vi "LaneExtractorHenes.vi"() -> ()   [LabVIEW 2024]
uses:
  <vilib>/userDefined/High Color/IMAQdx.ctl
  <vilib>/Instr/_visa.llb/VISA Set IO Buffer Mask.ctl
  <vilib>/Instr/_visa.llb/VISA Flush IO Buffer Mask.ctl
  <vilib>/Python/Open Venv Python Session.vi
  <vilib>/Instr/_visa.llb/VISA Configure Serial Port (Instr).vi
  <vilib>/vision/NI_Vision_Development_Module.lvlib
  <vilib>/vision/driver/NI_Vision_Acquisition_Software.lvlib
panel:
  in  "File Path":path=path "C:/Users/JungiHong/OneDrive/Hongik/HI-RACE/2026-01/ExperimentModules/LaneTracking/sampleImages/KakaoTalk_20260312_120930048.jpg"
  in  "UseVideo":bool
  in  "Cam No.":T1="cam3"
  out "Debug":T2(plugin-control)
  in  "input_spd":i16
  in  "HENES":refnum<visa-resource-name>="COM5"
  out "E-STOP":bool
  out "Remote_M/A":bool
  out "Steer_Feed":dbl
  out "Alive_PCU":u8(slide) scale=0.0..254.0
  out "Gear_Feed":u8
  out "Speed_Feed(RPM)":dbl format="%#_g rpm"
  out "버퍼 읽기":string
  out "Speed_Feed(m/s)":dbl
  in  "HLV_Gear":u8
  in  "HLV_A/M":bool=TRUE
  in  "HLV_E-stop":bool
  out "HENES Loop Time":u32=19
  in  "v(Velocity)m/s":dbl=1.0
  in  "k(Gain)":dbl=1.0
  out "δ(OutputSteer)degrees":dbl=17.662742890531817
  in  "max_rmse":u32=1000
  in  "min_span":u32=4
  in  "min_area":u32=4
  out "Right":T2(plugin-control)
  out "B":u8[][](array[numeric])
  out "G":u8[][](array[numeric])
  out "R":u8[][](array[numeric])
  out "changearray":u32=6
  out "CV Loop Time":u32=134
  out "error out 2":errorcluster
  out "error out":errorcluster
  out "return value":string[](array[string])=["0.0", "0.31842436928828866", "C:\\Users\\JungiHong\\OneDrive\\Hongik\\HI-RACE\\2026-01\\ExperimentModules\\LaneTracking\\DebugImageFolder\\left_lane.png", "C:\\Users\\JungiHong\\OneDrive\\Hongik\\HI-RACE\\2026-01\\ExperimentModules\\LaneTracking\\DebugImageFolder\\right_lane.png", "C:\\Users\\JungiHong\\OneDrive\\Hongik\\HI-RACE\\2026-01\\ExperimentModules\\LaneTracking\\DebugImageFolder\\debug_image.png"]
  out "python_error":errorcluster
  out "Left":T2(plugin-control)
  in  "stop":bool
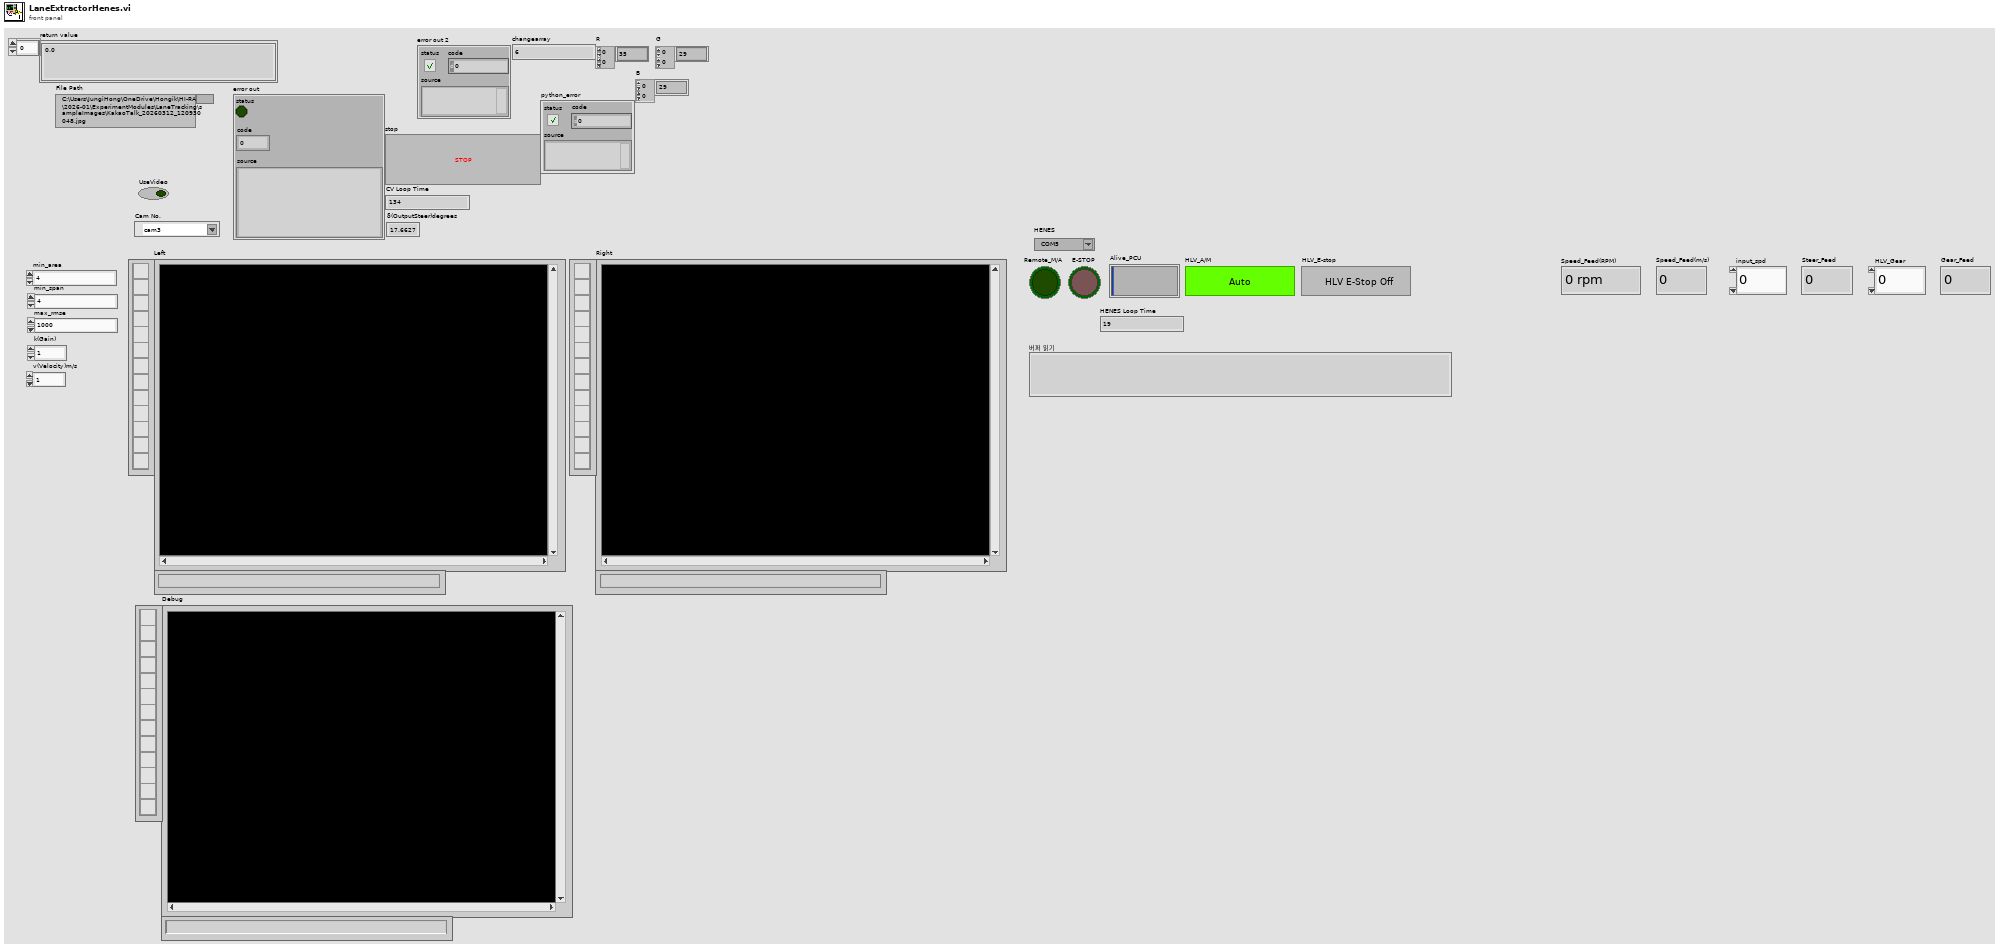
[diagram p1: front panel]
types:
  T1 = typedef "IMAQdx.ctl" = refnum<k21>
  T2 = typedef "IMAQ Image.ctl" = refnum<image>
  T3 = cluster{"HENES_M/A":u8, "HENES_E-Stop":u8, "HENES_Gear":u8, "HENES_Speed":i16, "HENES_Steer":i16, "HENES_Alive":u8}
  T4 = typedef "VISA Flush IO Buffer Mask.ctl" = u16
  T5 = typedef "VISA Set IO Buffer Mask.ctl" = u16
  T6 = cluster{"HLV_M/A_Status":u8, "HLV_E-Stop":u8, "HLV_Gear":u8, "HLV_Speed":i16, "HLV_Steer":i16, "HLV_Alive":u8}
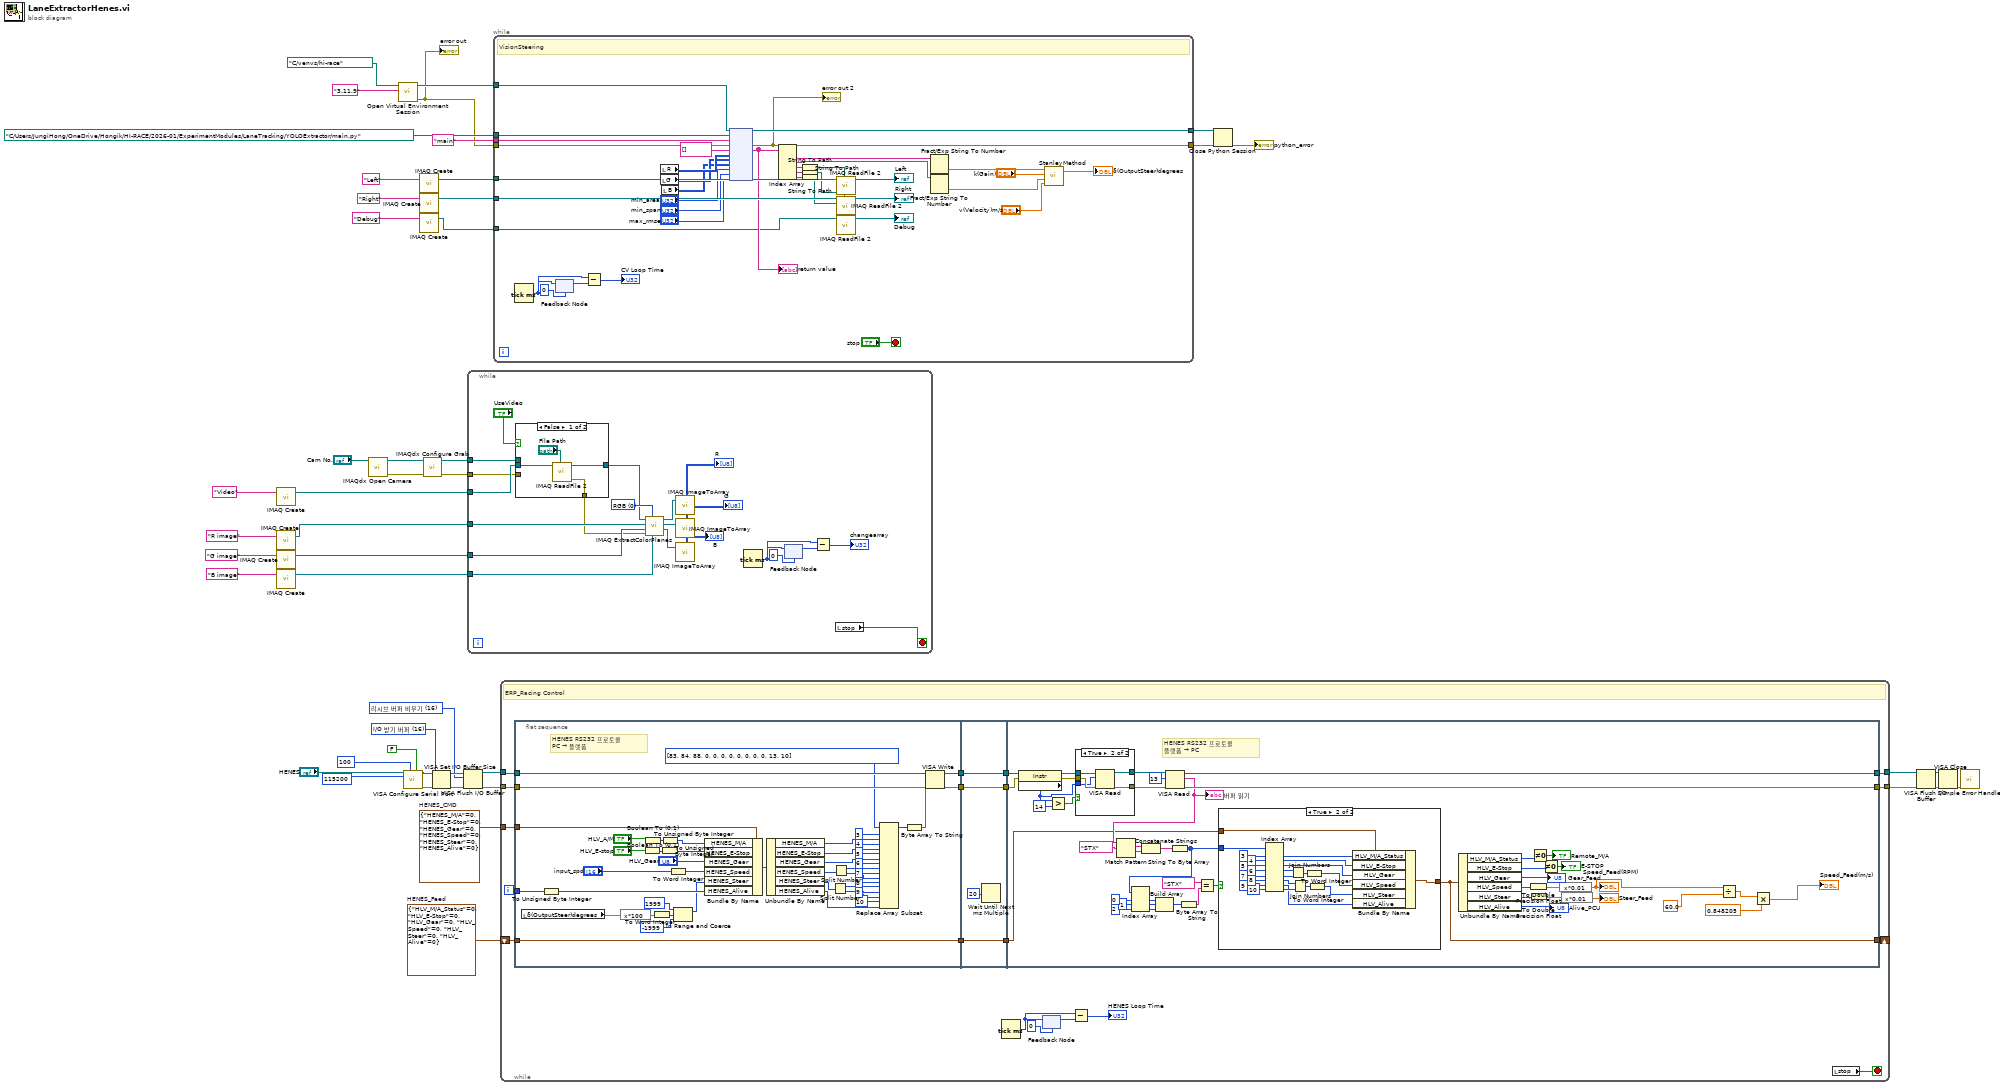
[diagram p0: block diagram]
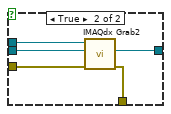
[diagram p4: hidden frame]
diagram:
  w9 = T3 {"HENES_M/A"=0, "HENES_E-Stop"=0, "HENES_Gear"=0, "HENES_Speed"=0, "HENES_Steer"=0, "HENES_Alive"=0}  # HENES_CMD
  w12 = T4 16 items=["리시브 버퍼 비우기"=16, "전달 버퍼 디바이스에 쓰기"=32, "리시브 버퍼 비우기(I/O 없음)"=64, "전달 버퍼 비우기"=128] ("Mask")
  w15 = T5 16 items=["I/O 받기 버퍼"=16, "I/O 전달 버퍼"=32, "I/O 받기와 전달 버퍼"=48] ("Mask")
  w19 = T6 {"HLV_M/A_Status"=0, "HLV_E-Stop"=0, "HLV_Gear"=0, "HLV_Speed"=0, "HLV_Steer"=0, "HLV_Alive"=0}  # HENES_Feed
  n1 = call "IMAQ Create"("Image Name"="Video") -> ("New Image"=w29:T2)  [unwired: 4 in, 1 out]
  n2 = call "IMAQ Create"("Image Name"="R image") -> ("New Image"=w30:T2)  [unwired: 4 in, 1 out]
  n3 = call "IMAQ Create"("Image Name"="G image") -> ("New Image"=w31:T2)  [unwired: 4 in, 1 out]
  n4 = call "IMAQ Create"("Image Name"="B image") -> ("New Image"=w32:T2)  [unwired: 4 in, 1 out]
  n5 = call <vilib>:"IMAQdx Open Camera.vi"("Session In"="Cam No.") -> ("error out"=w3:errorcluster, "Session Out"=w4:T1)  [unwired: 9 in]
  n6 = call-poly <vilib>:"Open Virtual Environment Session.vi"("Python version"="3.11.9", "Env path"=path "C:/venvs/hi-race") -> ("error out"=w37:errorcluster, "session out"=w47:refnum<k35>)  [unwired: 8 in]
  "error out" <- w37
  n7 = call-poly "VISA Configure Serial Port"("VISA resource name"="HENES", "timeout (10sec)"=u32 100, "Enable Termination\nChar (T)"=FALSE ("Enable Termination\nChar (T)"), "baud rate (9600)"=u32 115200) -> ("VISA resource name out"=w11:refnum<visa-resource-name>, "error out"=w10:errorcluster)  [unwired: 10 in]
  n8 = call "IMAQ Create"("Image Name"="Left") -> ("New Image"=w42:T2)  [unwired: 4 in, 1 out]
  n9 = call "IMAQ Create"("Image Name"="Right") -> ("New Image"=w27:T2)  [unwired: 4 in, 1 out]
  n10 = call "IMAQ Create"("Image Name"="Debug") -> ("New Image"=w6:T2)  [unwired: 4 in, 1 out]
  n11 = call <vilib>:"IMAQdx Configure Grab.vi"("error in"=w3, "Session In"=w4) -> ("error out"=w2:errorcluster, "Session Out"=w5:T1)  [unwired: 8 in]
  n12 = VISA Set I/O Buffer Size(VISA resource name=w11, mask (16)=w15, error in (no error)=w10) -> (VISA resource name out=w14:refnum<visa-resource-name>, error out=w13:errorcluster)  [unwired: 1 in]
  n13 = VISA Flush I/O Buffer(VISA resource name=w14, mask (16)=w12, error in (no error)=w13) -> (VISA resource name out=w24:refnum<visa-resource-name>, error out=w23:errorcluster)
  n14 = while {
    tunnel: w32 -> [w63]
    tunnel: w31 -> [w62]
    tunnel: w30 -> [w61]
    tunnel: w29 -> [w53]
    tunnel: w5 -> [w50]
    tunnel: w2 -> [w49]
    stop <- w68 stop-if-true
    w67 = u16 0 items=["RGB", "HSL", "HSV", "HSI"] ("Color Mode")
    n15 = case shown="False" "UseVideo" {
      tunnel: w53 -> [w70 w77]
      tunnel: [w72 w76] -> w52
      tunnel: [w71 w75] -> w51
      tunnel: w50 -> [_ w74]
      tunnel: w49 -> [_ w73]
      frame False {
        n16 = call "IMAQ ReadFile 2"("File Path"="File Path", "Image"=w70) -> ("error out"=w72:errorcluster, "Image Out"=w71:T2)  [unwired: 5 in, 3 out]
      }
      frame True {
        n17 = call <vilib>:"IMAQdx Grab2.vi"("error in"=w73, "Image In"=w77, "Session In"=w74) -> ("error out"=w76:errorcluster, "Image Out"=w75:T2)  [unwired: 5 in, 2 out]
      }
    }
    n18 = call "IMAQ ExtractColorPlanes"("Blue or Luma or Val or Inten Plane"=w63, "Color Mode"=w67, "error in (no error)"=w52, "Green or Sat Plane"=w62, "Red or Hue Plane"=w61, "Image Src"=w51) -> ("Blue or Luma or Val or Inten Plane out"=w64:T2, "Green or Sat Plane out"=w65:T2, "Red or Hue Plane out"=w66:T2)  [unwired: 2 in, 1 out]
    n19 = call "IMAQ ImageToArray"("Image"=w66) -> ("Image Pixels (U8)"=→"R":u8[][])  [unwired: 3 in, 4 out]
    n20 = call "IMAQ ImageToArray"("Image"=w65) -> ("Image Pixels (U8)"=→"G":u8[][])  [unwired: 3 in, 4 out]
    n21 = call "IMAQ ImageToArray"("Image"=w64) -> ("Image Pixels (U8)"=→"B":u8[][])  [unwired: 3 in, 4 out]
    n22 = Tick Count (ms)() -> (millisecond timer value=w57:u32)
    n23 = feedback #1(u32 0 ("millisecond timer value")) -> (w58:u32)
    n24 = feedback-in #1(w57) -> ()
    n25 = Subtract(x=w57, y=w58) -> (x-y=→"changearray":u32)
    n26 = local read "stop"() -> (w68:bool)
  }
  n27 = while {
    tunnel: w47 -> [w114]
    tunnel: [w113] -> w44
    tunnel: w42 -> [w107]
    tunnel: path "C:/Users/JungiHong/OneDrive/Hongik/HI-RACE/2026-01/ExperimentModules/LaneTracking/YOLOExtractor/main.py" ("module in") -> [w111]
    tunnel: "main" ("module out") -> [w110]
    tunnel: w37 -> [w109]
    tunnel: [w108] -> w39
    tunnel: w27 -> [w96]
    tunnel: w6 -> [w78]
    stop <- "stop" stop-if-true
    # "VisionSteering"
    n28 = Tick Count (ms)() -> (millisecond timer value=w104:u32)
    n29 = feedback #2(u32 0 ("millisecond timer value")) -> (w103:u32)
    n30 = feedback-in #2(w104) -> ()
    n31 = Subtract(x=w104, y=w103) -> (x-y=→"CV Loop Time":u32)
    n32 = local read "G"() -> (w99:u8[][])
    n33 = local read "R"() -> (w100:u8[][])
    n34 = local read "B"() -> (w98:u8[][])
    n35 = node(w114, w111, w110, w109, string[] [], w100, w99, w98, "min_area", "min_span", "max_rmse") -> (w113:refnum<k35>, w108:errorcluster, w95:string[])  [unwired: 6 in, 2 out]
    "return value" <- w95
    "error out 2" <- w108
    n36 = Index Array(array=w95) -> (element #1=w88:string, element #2=w87:string, element #3=w90:string, element #4=w89:string, element #5=w80:string)  [unwired: 5 in]
    n37 = String To Path(string=w90) -> (path=w105:path)
    n38 = String To Path(string=w89) -> (path=w94:path)
    n39 = String To Path(string=w80) -> (path=w79:path)
    n40 = call "IMAQ ReadFile 2"("File Path"=w105, "Image"=w107) -> ("Image Out"=→"Left":T2)  [unwired: 5 in, 4 out]
    n41 = call "IMAQ ReadFile 2"("File Path"=w94, "Image"=w96) -> ("Image Out"=→"Right":T2)  [unwired: 5 in, 4 out]
    n42 = call "IMAQ ReadFile 2"("File Path"=w79, "Image"=w78) -> ("Image Out"=→"Debug":T2)  [unwired: 5 in, 4 out]
    n43 = Fract/Exp String To Number(string=w88) -> (number=w85:dbl)  [unwired: 3 in, 1 out]
    n44 = Fract/Exp String To Number(string=w87) -> (number=w84:dbl)  [unwired: 3 in, 1 out]
    n45 = call "StanleyMethod.vi"("v(Velocity)m/s"="v(Velocity)m/s", "e(Cross-Track Err)m/s"=w84, "k(Gain)"="k(Gain)", "ψ(Heading Err)radian"=w85) -> ("δ(OutputSteer)degrees"=→"δ(OutputSteer)degrees":dbl)  [unwired: 1 out]
  }
  n46 = while {
    tunnel: w24 -> [w134]
    tunnel: w23 -> [w133]
    tunnel: [w127] -> w22
    tunnel: [w126] -> w21
    shift-right: [w121] -> _
    shift-left: w19 -> [w124]
    tunnel: w9 -> [w122]
    i -> [w128]
    stop <- w116 stop-if-true
    # "ERP_Racing Control"
    n47 = flat-sequence {
      tunnel: [w177] -> w131
      tunnel: [w176] -> w129
      tunnel: w134 -> [w179]
      tunnel: w133 -> [w178]
      tunnel: w128 -> [w175]
      tunnel: [w174] -> w125
      tunnel: w124 -> [w174]
      tunnel: w122 -> [w173]
      tunnel: [w183] -> w132
      tunnel: w131 -> [w183]
      tunnel: [w182] -> w130
      tunnel: w129 -> [w182]
      tunnel: w125 -> [w180]
      tunnel: [w180] -> w123
      tunnel: w132 -> [w211]
      tunnel: w130 -> [w210]
      tunnel: [w228] -> w127
      tunnel: [w227] -> w126
      tunnel: w123 -> [w202]
      tunnel: [w200] -> w121
      frame #0 {
        # "HENES RS232 프로토콜\nPC → 플랫폼"
        n48 = local read "δ(OutputSteer)degrees"() -> (w135:dbl)
        n49 = To Unsigned Byte Integer(number=w175) -> (unsigned 8bit integer=w162:u8)
        n50 = expression code="x*100"(w135) -> (w137:dbl)
        n51 = Boolean To (0,1)(Boolean="HLV_E-stop") -> (0, 1=w157:i16)
        n52 = Boolean To (0,1)(Boolean="HLV_A/M") -> (0, 1=w158:i16)
        n53 = To Word Integer(number=w137) -> (16bit integer=w140:i16)
        n54 = To Unsigned Byte Integer(number=w157) -> (unsigned 8bit integer=w155:u8)
        n55 = To Unsigned Byte Integer(number=w158) -> (unsigned 8bit integer=w156:u8)
        n56 = To Word Integer(number="input_spd") -> (16bit integer=w149:i16)
        n57 = In Range and Coerce(upper limit=i16 1999 ("상위 리미트"), x=w140, lower limit=i16 -1999 ("상위 리미트")) -> (coerced(x)=w148:i16)  [unwired: 1 out]
        n58 = Bundle By Name(cluster=w173, "HENES_M/A"=w156, "HENES_E-Stop"=w155, "HENES_Gear"="HLV_Gear", "HENES_Speed"=w149, "HENES_Steer"=w148, "HENES_Alive"=w162) -> (w166:T3)
        n59 = Unbundle By Name(w166) -> ("HENES_M/A"=w152:u8, "HENES_E-Stop"=w151:u8, "HENES_Gear"=w141:u8, "HENES_Speed"=w144:i16, "HENES_Steer"=w147:i16, "HENES_Alive"=w161:u8)
        n60 = Split Number(x=w147) -> (hi(x)=w146:u8, lo(x)=w145:u8)
        n61 = Split Number(x=w144) -> (hi(x)=w143:u8, lo(x)=w142:u8)
        n62 = Replace Array Subset(array=u8[] [83, 84, 88, 0, 0, 0, 0, 0, 0, 0, 0, 13, 10] ("unsigned byte array"), new element #1=w152, index #1=3, new element #2=w151, index #2=4, new element #3=w141, index #3=5, new element #4=w143, index #4=6, new element #5=w142, index #5=7, new element #6=w146, index #6=8, new element #7=w145, index #7=9, new element #8=w161, index #8=10) -> (w164:u8[])
        n63 = Byte Array To String(unsigned byte array=w164) -> (string=w163:string)
        n64 = VISA Write(VISA resource name=w179, write buffer=w163, error in (no error)=w178) -> (VISA resource name out=w177:refnum<visa-resource-name>, error out=w176:errorcluster)  [unwired: 1 out]
      }
      frame #1 {
        n65 = Wait Until Next ms Multiple(millisecond multiple=u32 20 ("대기 시간 (ms)")) -> ()  [unwired: 1 out]
      }
      frame #2 {
        # "HENES RS232 프로토콜\n플랫폼 → PC"
        n66 = property class="Instr"(reference=w211, error in=w210) -> (reference out=w191:refnum<visa-resource-name>, error out=w190:errorcluster, "Serial Settings:Number of Bytes at Serial Port"=w189:u32)
        n67 = Greater?(x=w189, y=u32 14) -> (0:w207:bool)
        n68 = case shown="True" w207 {
          tunnel: w191 -> [w255 w260]
          tunnel: w190 -> [w254 w259]
          tunnel: [w255 w258] -> w209
          tunnel: [w254 w257] -> w208
          tunnel: w189 -> [_ w256]
          frame False {
          }
          frame True {
            n69 = VISA Read(VISA resource name=w260, byte count=w256, error in (no error)=w259) -> (VISA resource name out=w258:refnum<visa-resource-name>, error out=w257:errorcluster)  [unwired: 2 out]
          }
        }
        n70 = VISA Read(VISA resource name=w209, byte count=u32 13, error in (no error)=w208) -> (VISA resource name out=w228:refnum<visa-resource-name>, read buffer=w226:string, error out=w227:errorcluster)  [unwired: 1 out]
        "버퍼 읽기" <- w226
        n71 = Match Pattern(string=w226, regular expression="STX") -> (match substring=w223:string, after substring=w224:string)  [unwired: 1 in, 2 out]
        n72 = Concatenate Strings(w223, w224) -> (w222:string)
        n73 = String To Byte Array(string=w222) -> (unsigned byte array=w204:u8[])
        n74 = Index Array(array=w204, index #1=0, index #2=1, index #3=2) -> (element #1=w217:u8, element #2=w216:u8, element #3=w215:u8)
        n75 = Build Array(w217, w216, w215) -> (w214:u8[])
        n76 = Byte Array To String(unsigned byte array=w214) -> (string=w212:string)
        n77 = Equal?(x="STX", y=w212) -> (x = y?=w203:bool)
        n78 = case shown="True" w203 {
          tunnel: w204 -> [_ w253]
          tunnel: [w230 w240] -> w200
          tunnel: w202 -> [w230 w242]
          frame False {
          }
          frame True {
            n79 = Index Array(array=w253, index #1=3, index #2=4, index #3=5, index #4=6, index #5=7, index #6=8, index #7=9, index #8=10) -> (element #1=w241:u8, element #2=w239:u8, element #3=w238:u8, element #4=w237:u8, element #5=w236:u8, element #6=w234:u8, element #7=w233:u8, element #8=w231:u8)
            n80 = Join Numbers(hi=w237, lo=w236) -> ((hi.lo)=w244:u16)
            n81 = Join Numbers(hi=w234, lo=w233) -> ((hi.lo)=w243:u16)
            n82 = To Word Integer(number=w244) -> (16bit integer=w235:i16)
            n83 = To Word Integer(number=w243) -> (16bit integer=w232:i16)
            n84 = Bundle By Name(cluster=w242, "HLV_M/A_Status"=w241, "HLV_E-Stop"=w239, "HLV_Gear"=w238, "HLV_Speed"=w235, "HLV_Steer"=w232, "HLV_Alive"=w231) -> (w240:T6)
          }
        }
        n85 = Unbundle By Name(w200) -> ("HLV_M/A_Status"=w201:u8, "HLV_E-Stop"=w195:u8, "HLV_Gear"=→"Gear_Feed":u8, "HLV_Speed"=w193:i16, "HLV_Steer"=w192:i16, "HLV_Alive"=→"Alive_PCU":u8)
        n86 = To Double Precision Float(number=w193) -> (double precision float=w205:dbl)
        n87 = To Double Precision Float(number=w192) -> (double precision float=w198:dbl)
        n88 = Not Equal To 0?(x=w201) -> (x != 0?=→"Remote_M/A":bool)
        n89 = Not Equal To 0?(x=w195) -> (x != 0?=→"E-STOP":bool)
        n90 = expression code="x*0.01"(w205) -> (w184:dbl)
        "Speed_Feed(RPM)" <- w184
        n91 = expression code="x*0.01"(w198) -> (→"Steer_Feed":dbl)
        n92 = Divide(x=w184, y=60.0) -> (x/y=w188:dbl)
        n93 = Multiply(x=w188, y=0.848205) -> (x*y=→"Speed_Feed(m/s)":dbl)
      }
    }
    n94 = Tick Count (ms)() -> (millisecond timer value=w118:u32)
    n95 = feedback #3(u32 0 ("millisecond timer value")) -> (w119:u32)
    n96 = feedback-in #3(w118) -> ()
    n97 = Subtract(x=w118, y=w119) -> (x-y=→"HENES Loop Time":u32)
    n98 = local read "stop"() -> (w116:bool)
  }
  n99 = Close Python Session(session in=w44, error in=w39) -> (11:→"python_error":errorcluster)
  n100 = VISA Flush I/O Buffer(VISA resource name=w22, error in (no error)=w21) -> (VISA resource name out=w25:refnum<visa-resource-name>, error out=w26:errorcluster)  [unwired: 1 in]
  n101 = VISA Close(VISA resource name=w25, error in (no error)=w26) -> (error out=w20:errorcluster)
  n102 = call <vilib>:"Simple Error Handler.vi"("error in (no error)"=w20) -> ()  [unwired: 4 in, 5 out]
